vi "emi_SMLoop Link loops.vi"(7 "Loop IDS":u16[](array[numeric]), 11 "error in (no error)":errorcluster) -> (15 "error out":errorcluster)   [LabVIEW 2011]
doc: "Check wheter a loop should start. based on loop enable(Loop control),\n\nExecutes as normal on error"
uses:
  Loop control/Private/_emi_Loop control int action.ctl
  Loop control/Private/_emi_GFV Loop Running.vi
  Private/_emi_ SMLoop Restart Counter.vi
  Loop control/Private/_emi_GFV stop a loop so it can reset.vi
  Private/_emi_ SMLoop Restart.vi
  Loop control/Private/_emi_GFV Loop Enable.vi
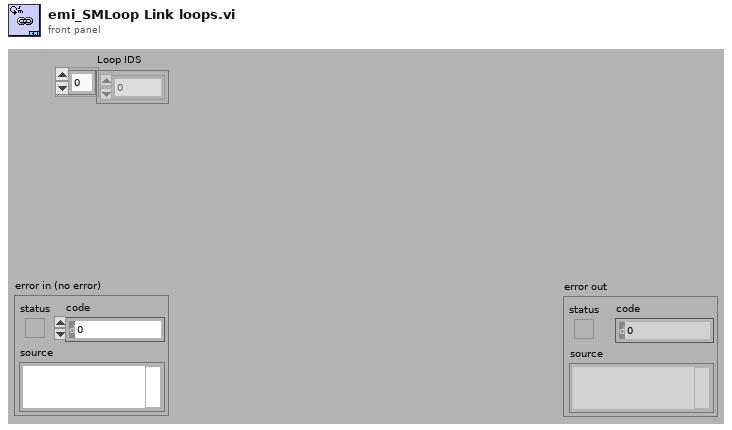
[diagram p1: front panel]
types:
  T1 = typedef "_emi_Loop control int action.ctl" = enum16{"Init index", "Get index", "Set index", "Get Size"}
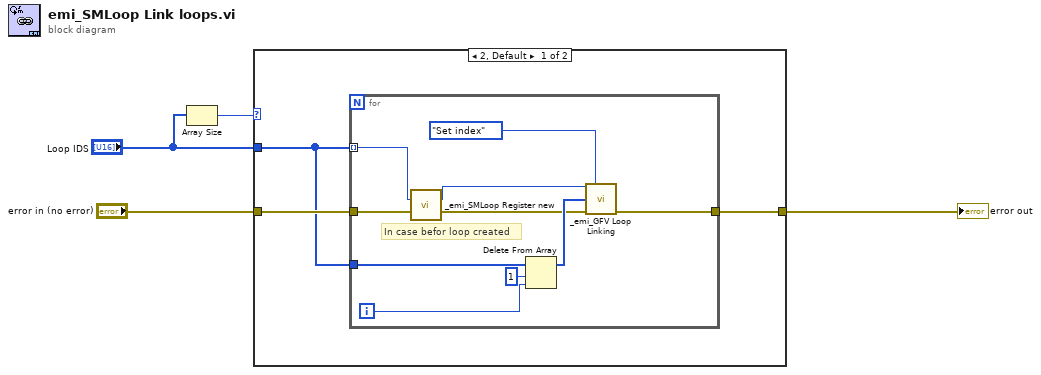
[diagram p0: block diagram]
diagram:
  n1 = Array Size(array="Loop IDS") -> (size(s)=w2:i32)
  n2 = case shown="2, Default" w2 {
    tunnel: "error in (no error)" -> [w7 w18]
    tunnel: [w5 w18] -> w3
    tunnel: "Loop IDS" -> [w6 _]
    frame 2, Default {
      n3 = for {
        tunnel: w7 -> [w11]
        tunnel: w6 -> [w10] mode=indexing
        tunnel: w6 -> [w14]
        tunnel: [w12] -> w5
        i -> [w15]
        # "In case befor loop created"
        n4 = call "_emi_SMLoop Register new.vi"("Loop ID"=w10, "error in (no error)"=w11) -> ("Loop ID Out"=w9:u16, "error out"=w8:errorcluster)  [unwired: 12 in]
        n5 = Delete From Array(array=w14, length=1, index=w15) -> (array with subset deleted=w13:u16[])  [unwired: 1 out]
        n6 = call "_emi_GFV Loop Linking.vi"("Loop Index/Numb"=w9, "Action(Get Index)"=_emi_Loop_control_int_action."Set index", "Linked indexes in"=w13, "error in (no error)"=w8) -> ("error out"=w12:errorcluster)  [unwired: 8 in, 3 out]
      }
    }
    frame 0, 1 {
      # "Intet å linke"
    }
  }
  "error out" <- w3
